vi "calcula_dora.vi"(9 "x":dbl, 10 "Mot_Min":dbl=0.35, 11 "Mot_Max":dbl=0.35) -> (1 "x+y":dbl)   [LabVIEW 2020]
panel:
  out "Negar":bool
  out "Lime_Max":dbl=0.35
  out "Lime_Min":dbl=0.35
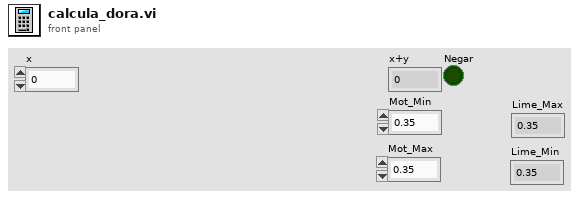
[diagram p1: front panel]
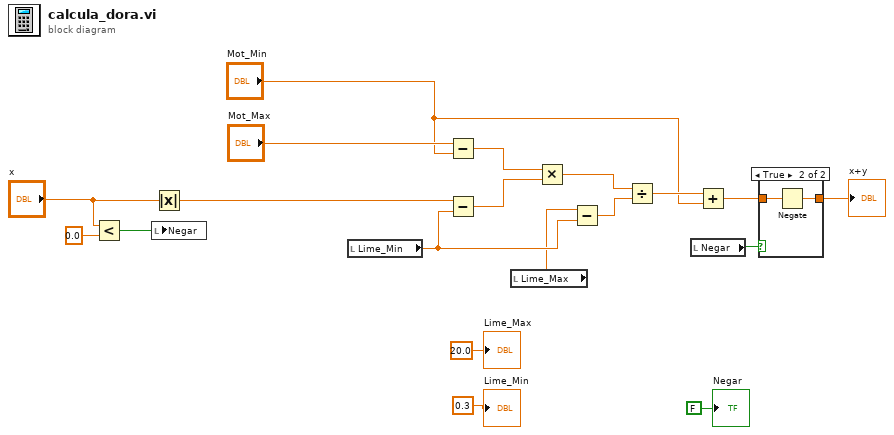
[diagram p0: block diagram]
diagram:
  n1 = Less?(x="x", y=0.0) -> (x < y?=w8:bool)
  n2 = local write "Negar"(w8) -> ()
  n3 = Absolute Value(x="x") -> (abs(x)=w6:dbl)
  n4 = local read "Lime_Min"() -> (w12:dbl)
  n5 = Subtract(x="Mot_Max", y="Mot_Min") -> (x-y=w19:dbl)
  n6 = Subtract(x=w6, y=w12) -> (x-y=w18:dbl)
  n7 = local read "Lime_Max"() -> (w11:dbl)
  n8 = Multiply(x=w19, y=w18) -> (x*y=w17:dbl)
  n9 = Subtract(x=w11, y=w12) -> (x-y=w16:dbl)
  n10 = Divide(x=w17, y=w16) -> (x/y=w15:dbl)
  n11 = local read "Negar"() -> (w5:bool)
  n12 = Add(x=w15, y="Mot_Min") -> (x+y=w4:dbl)
  n13 = case shown="True" w5 {
    tunnel: w4 -> [w20 w22]
    tunnel: [w20 w21] -> w3
    frame False {
    }
    frame True {
      n14 = Negate(x=w22) -> (-x=w21:dbl)
    }
  }
  "x+y" <- w3
  "Lime_Max" <- 20.0 ("x")
  "Lime_Min" <- 0.3 ("x")
  "Negar" <- FALSE
